vi "Configure Hardware.vi"(8 "error in (no error)":errorcluster, 11 "Hardware Resources in":T1={"Test Setting"={"Test_Num"=0, "Test_ID"=0, "Proc_ID"=0, "Max Force"=0.0, "User"="", "SN"="", "Date"=""}, "Measurements"=[[""]], "LOG REF"=refnum, "Report Template"=path "", "Save Report path"=path "", "Data File Path"=path "", "Popup Dialog"=FALSE}) -> (0 "error out":errorcluster, 3 "Hardware Resources out":T1)   [LabVIEW 2020, in "Report.lvlib"]
doc: "Configure the hardware."
uses:
  Report.lvlib
  REP Configuration.ctl
  Test Setting.ctl
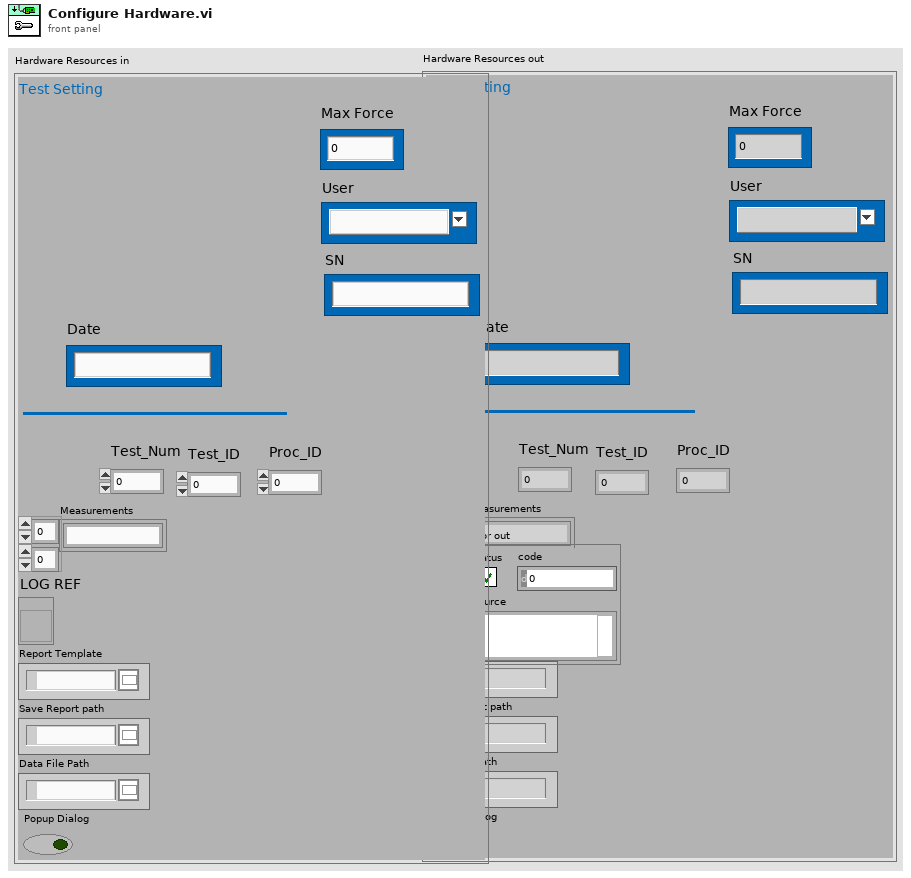
[diagram p1: front panel]
types:
  T1 = typedef "Report.lvlib/REP Configuration.ctl" = cluster{"Test Setting":T2, "Measurements":string[][], "LOG REF":refnum<vi>, "Report Template":path, "Save Report path":path, "Data File Path":path, "Popup Dialog":bool}
  T2 = typedef "Report.lvlib/Test Setting.ctl" = cluster{"Test_Num":i32, "Test_ID":i32, "Proc_ID":i32, "Max Force":dbl, "User":string, "SN":string, "Date":string}
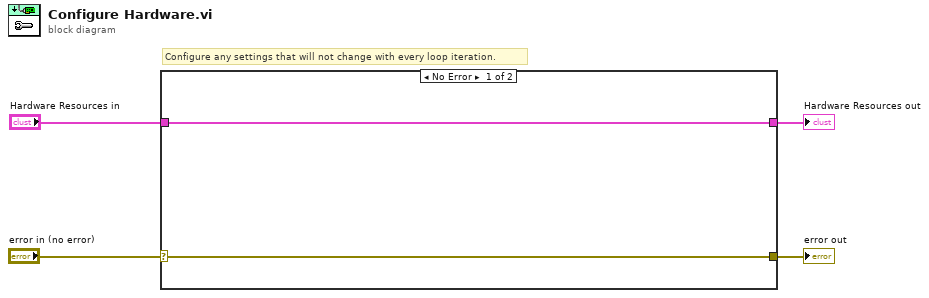
[diagram p0: block diagram]
diagram:
  # "Configure any settings that will not change with every loop iteration."
  n1 = case shown="No Error" "error in (no error)" {
    selector: "error in (no error)" -> [w6 w7]
    tunnel: [w6 w7] -> w3
    tunnel: "Hardware Resources in" -> [w5 w8]
    tunnel: [w5 w8] -> w1
    frame No Error {
    }
    frame Error {
    }
  }
  "Hardware Resources out" <- w1
  "error out" <- w3
